vi "Launcher.vi"   [LabVIEW 2019]
uses:
  Actors/TopLevel/TopLevel/TopLevel.lvclass
  C:/Program Files/National Instruments/LabVIEW 2019/vi.lib/ActorFramework/Actor/Actor.lvclass
  Actors/TopLevel/TopLevel Messages/Load Msg/Load Msg.lvclass/Load Msg.ctl
  <vilib>/ActorFramework/Message Enqueuer/Message Enqueuer.lvclass/Message Enqueuer.ctl
  <vilib>/ActorFramework/Message Enqueuer/Enqueue.vi
  Actors/TopLevel/TopLevel Messages/Load Msg/Load Msg.lvclass
  C:/Program Files/National Instruments/LabVIEW 2019/vi.lib/ActorFramework/Message/Message.lvclass
  <vilib>/ActorFramework/Stop Msg/Stop Msg.lvclass
  <vilib>/ActorFramework/Message Priority Queue/Priority Enqueue.vi
  <vilib>/ActorFramework/Actor/Actor.lvclass
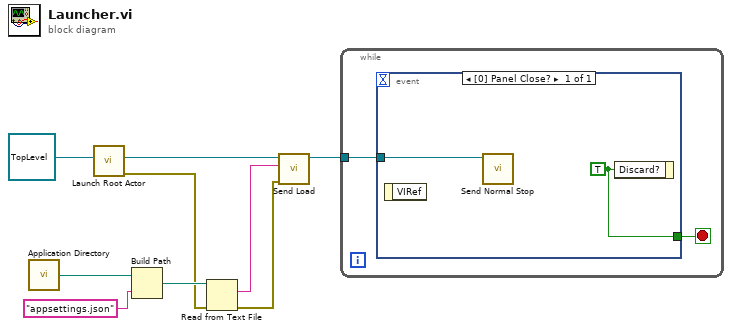
[diagram p0: block diagram]
diagram:
  n1 = call <vilib>:"Application Directory.vi"() -> ("Application Directory"=w6:path)
  n2 = call <vilib>:"Launch Root Actor.vi"("Actor"=refnum<class "TopLevel.lvclass"> refnum ("TopLevel.lvlib:TopLevel.lvclass")) -> ("error out"=w3:errorcluster, "Actor's Enqueuer"=w8:refnum<class "Message Enqueuer.lvclass">)  [unwired: 9 in]
  n3 = Build Path(base path=w6, name or relative path="appsettings.json") -> (appended path=w4:path)
  n4 = Read from Text File(file (use dialog)=w4, error in=w3) -> (text=w1:string, error out=w2:errorcluster)  [unwired: 2 in, 2 out]
  n5 = call "Send Load.vi"("error in (no error)"=w2, "JSON"=w1, "Message Enqueuer"=w8) -> ("Message Enqueuer out"=w7:refnum<class "Message Enqueuer.lvclass">)  [unwired: 7 in, 1 out]
  n6 = while {
    tunnel: w7 -> [w10]
    stop <- w11 stop-if-true
    n7 = event shown="[0] Panel Close?" {
      selector: _ -> [_]
      dyn-events: _ -> [_]
      timeout: _ -> [_]
      tunnel: [w13] -> w11
      tunnel: w10 -> [w12]
      event Panel Close? {
        w13 = TRUE ("Discard?")
        n8 = event-data() -> ()  [unwired: 1 in, 1 out]
        n9 = call <vilib>:"Send Normal Stop.vi"("Message Enqueuer"=w12) -> ()  [unwired: 10 in, 1 out]
        n10 = event-data("Discard?"=w13) -> ()  [unwired: 1 in, 1 out]
      }
    }
  }
